vi "Read Measurement 2 Channels.vi"(8 "error in (no error)":errorcluster, 10 "Parameters":T1={"Channel 1 (1: Channel 1)"=1, "Channel 2 (2: Channel 2)"=2, "Measurement Type (0: Phase)"=0} {"Measurement Type (0: Phase)" items=["Phase", "Delay", "DelayRR", "DelayRF", "DelayFR", "DelayFF"]; "Channel 2 (2: Channel 2)" items=["Channel 1"=1, "Channel 2"=2, "Channel 3"=3, "Channel 4"=4]; "Channel 1 (1: Channel 1)" items=["Channel 1"=1, "Channel 2"=2, "Channel 3"=3, "Channel 4"=4]}, 11 "Tektonix 2000 in":refnum<class "Tektonix 2000.lvclass">) -> (0 "error out":errorcluster, 1 "Units":string, 2 "Measurement":dbl, 3 "Tektonix 2000 out":refnum<class "Tektonix 2000.lvclass">)   [LabVIEW 2020, in "Osciloscope Tektronix.lvlib" / "Tektonix 2000.lvclass"]
uses:
  Tektonix 2000.lvclass
  C:/Users/Pablo/Osciloscope-Tek/TDS2000/Libraries/Osciloscope Tektronix/Clases/Osciloscope/Osciloscope.lvclass
  Osciloscope/Osciloscope.lvclass/Osciloscope.ctl
  Osciloscope/Read COM.vi
  <instrlib>/Tektronix TDS 200 1000 2000 Series/Tektronix TDS 200 1000 2000 Series.lvlib
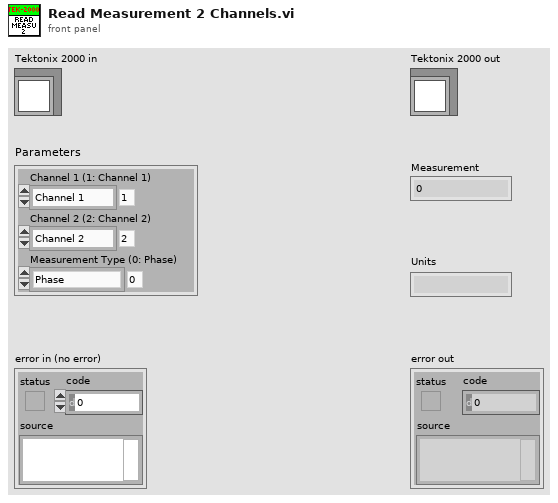
[diagram p1: front panel]
types:
  T1 = cluster{"Channel 1 (1: Channel 1)":i32, "Channel 2 (2: Channel 2)":i32, "Measurement Type (0: Phase)":i32}
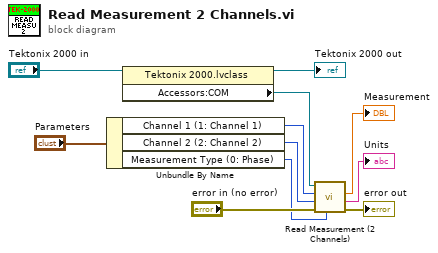
[diagram p0: block diagram]
diagram:
  n1 = Unbundle By Name("Parameters") -> ("Channel 1 (1: Channel 1)"=w3:i32, "Channel 2 (2: Channel 2)"=w2:i32, "Measurement Type (0: Phase)"=w1:i32)
  n2 = property class="Tektonix 2000.lvclass"(reference="Tektonix 2000 in") -> (reference out=→"Tektonix 2000 out":refnum<class "Tektonix 2000.lvclass">, "Accessors:COM"=w5:refnum<visa-resource-name>)  [unwired: 1 in, 1 out]
  n3 = call <instrlib>:"Read Measurement (2 Channels).vi"("Measurement Type (0: Phase)"=w1, "error in (no error)"="error in (no error)", "Channel 2 (2: Channel 2)"=w2, "Channel 1 (1: Channel 1)"=w3, "VISA resource name"=w5) -> ("error out"=→"error out":errorcluster, "Units"=→"Units":string, "Measurement"=→"Measurement":dbl)  [unwired: 3 in, 1 out]
